vi "Read configuration.vi"(8 "error in":errorcluster, 11 "Simple Sequencer TBM editor node in":refnum<class "Simple Sequencer TBM editor node.lvclass">) -> (0 "error out":errorcluster, 2 "configuration":refnum<class "NISE_CEF_serializable configuration.lvclass">, 3 "Simple Sequencer TBM editor node out":refnum<class "Simple Sequencer TBM editor node.lvclass">)   [LabVIEW 2014, in "Simple Sequencer TBM editor node.lvclass"]
uses:
  Simple Sequencer TBM editor node.lvclass
  <vilib>/NI/Configuration Framework/serializable configuration/NISE_CEF_serializable configuration.lvclass
  Simple Sequencer TBM editor node.lvclass/Simple Sequencer TBM editor node.ctl
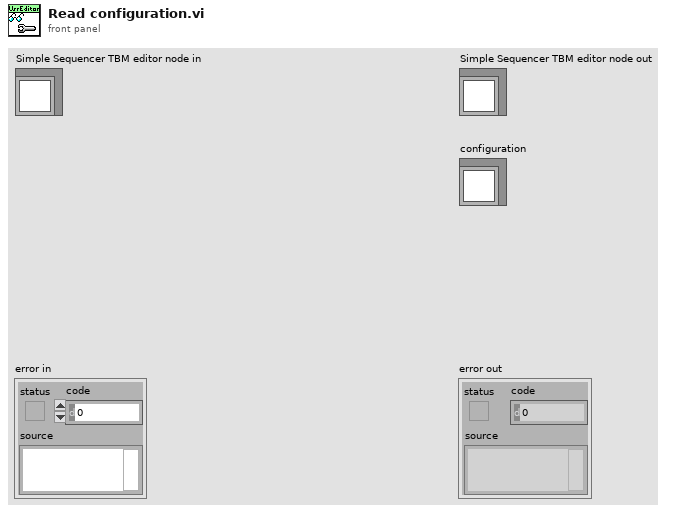
[diagram p1: front panel]
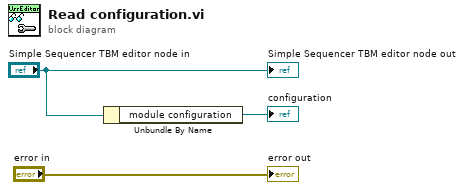
[diagram p0: block diagram]
diagram:
  n1 = Unbundle By Name("Simple Sequencer TBM editor node in") -> ("module configuration"=→"configuration":refnum<class "Simple Sequencer TBM configuration.lvclass">)
  "error out" <- "error in"
  "Simple Sequencer TBM editor node out" <- "Simple Sequencer TBM editor node in"
